vi "Search New Tweets - Continuous.vi"() -> ()   [LabVIEW 2011]
uses:
  Controls/Tweet.ctl
  i3-twitter.lvlib
panel:
  in  "Query":string
  in  "Consumer Secret":string
  in  "Consumer Key":string
  in  "Num of Tweets to Read":i32
  out "Num of Tweets Read":i32
  out "Time Stamp of Newest Tweet":timestamp
  in  "stop":bool
  out "Tweets Read":T1[](array[typedef])
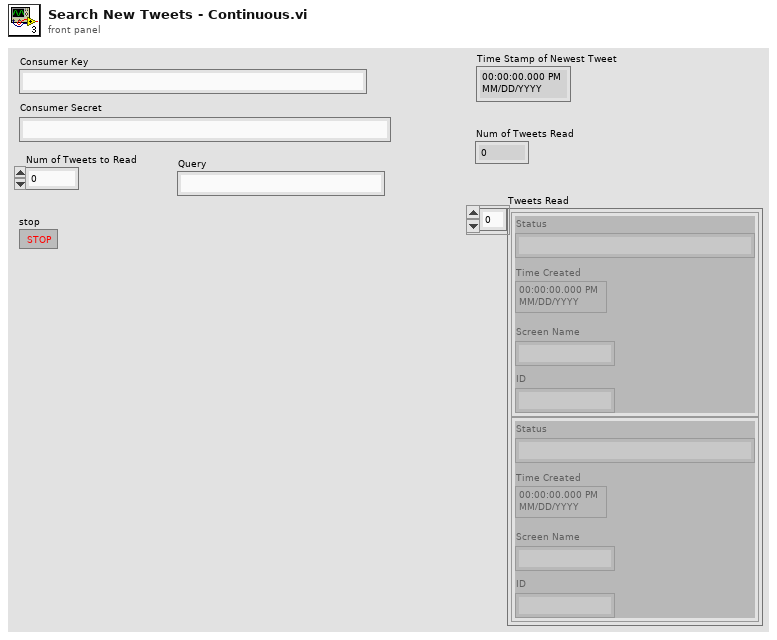
[diagram p1: front panel]
types:
  T1 = typedef "i3-twitter.lvlib/Tweet.ctl" = cluster{"Status":string, "Time Created":timestamp, "Screen Name":string, "ID":string}
  T2 = typedef "i3-oauth.lvlib/Credentials.ctl" = cluster{"Token":string, "Secret":string}
  T3 = typedef "i3-twitter.lvlib/Twitter Handle.ctl" = cluster{"OAuth Credentials":T4, "since ID":string, "max ID":string, "Screen Name":string}
  T4 = typedef "i3-oauth.lvlib/OAuth Handle.ctl" = cluster{"Signature Method":T5, "Version":string, "Client":T2, "Access":T2}
  T5 = typedef "i3-oauth.lvlib/Signature Method.ctl" = enum16{"HMAC-MD5", "HMAC-SHA1", "HMAC-SHA224", "HMAC-SHA256", "HMAC-SHA384", "HMAC-SHA512"}
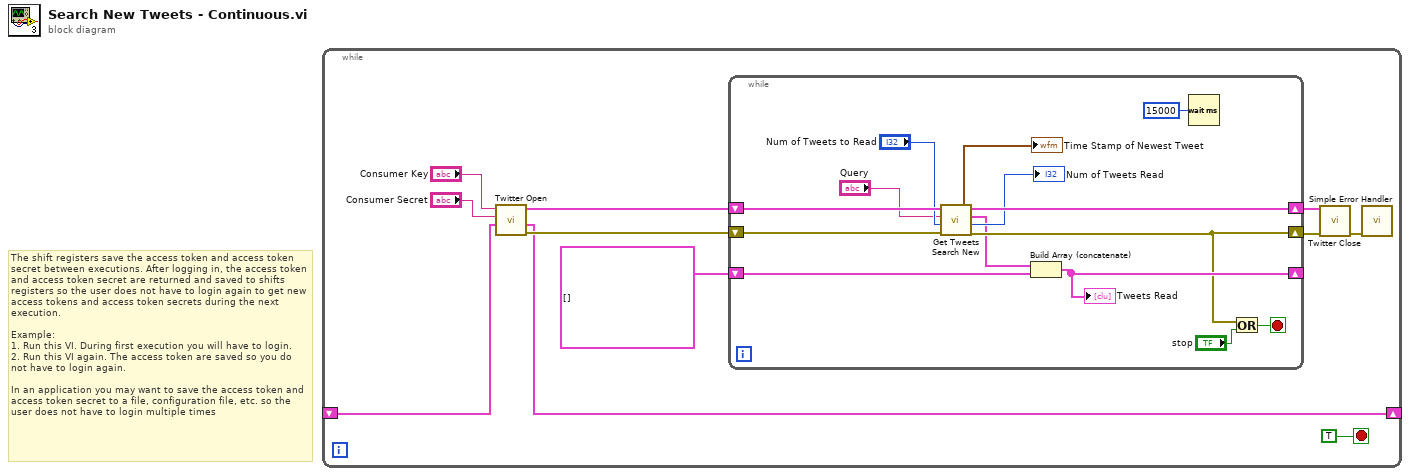
[diagram p0: block diagram]
diagram:
  # "The shift registers save the access token and access token secret between executions. After logging in, the access token and access token secret are returned and saved to shifts registers so the user does not have to login again to get new access tokens and access token secrets during the next execution.\n\nExample:\n1. Run this VI. During first execution you will have to login.\n2. Run this VI again. The access token are saved so you do not have to login again.\n\nIn an application you may want to save the access token and access token secret to a file, configuration file, etc. so the user does not have to login multiple times"
  n1 = while {
    shift-right: [w2] -> _
    shift-left: _ -> [w1]
    stop <- TRUE stop-if-true
    n2 = call "Twitter Open.vi"("Access Credentials (in)"=w1, "Consumer Secret"="Consumer Secret", "Consumer Key"="Consumer Key") -> ("error out"=w5:errorcluster, "Access Credentials (out)"=w2:T2, "Twitter Handle Out"=w9:T3)  [unwired: 6 in]
    n3 = while {
      shift-right: [w23] -> w7
      shift-left: w9 -> [w25]
      shift-right: [w21] -> _
      shift-left: T1[] [] ("Tweets Array") -> [w14]
      shift-right: [w18] -> w8
      shift-left: w5 -> [w24]
      stop <- w17 stop-if-true
      n4 = call "Get Tweets Search New.vi"("error in"=w24, "Tweets to Read (10)"="Num of Tweets to Read", "Query"="Query", "Twitter Handle In"=w25) -> ("error out"=w18:errorcluster, "Actual Num of Tweets Read"=→"Num of Tweets Read":i32, "New Tweets Read"=w15:T1[], "Twitter Handle Out"=w23:T3, "Time Stamp of Newest Tweet"=→"Time Stamp of Newest Tweet":timestamp)  [unwired: 3 in]
      n5 = Build Array (concatenate)(w15, w14) -> (w21:T1[])
      "Tweets Read" <- w21
      n6 = Wait (ms)(milliseconds to wait=u32 15000) -> ()  [unwired: 1 out]
      n7 = Or(x=w18, y="stop") -> (x .or. y?=w17:bool)
    }
    n8 = call "Twitter Close.vi"("error in"=w8, "Twitter Handle In"=w7) -> ("error in"=w3:errorcluster)  [unwired: 9 in]
    n9 = call <vilib>:"Simple Error Handler.vi"("error in (no error)"=w3) -> ()  [unwired: 4 in, 5 out]
  }
